vi "create_save_log_file.vi"(0 "Username":string, 1 "Data filepath":path, 2 "Frequency (Hz)":string="280", 3 "Application Directory":string, 5 "Experiment Title":string, 7 "Time constant (ms)":string="100 ms", 9 "Device details":T2={"Device label"="", "Experiment Variable"="", "Variable Value"="", "Pixel"=enum."1"}, 11 "Measurement settings":T1={"Start Wavelength (nm)"=300.0, "End Wavelength (nm)"=900.0, "Increment (nm)"=5.0, "White Bias (No. of Suns)"=1.0, "Averages per wavlength"=1.0, "Time Constant"=8, "Low Pass Filter Slope "=1, "Gain (V/A)"=50.0} {"Gain (V/A)" format="%#.2f"; "Low Pass Filter Slope" items=["6 dB/oct", "12 dB/oct", "18 db/oct", "24 dB/oct"]; "Time Constant" items=["10 us", "30 us", "100 us", "300 us", "1 ms", "3 ms", "10 ms", "30 ms", "100 ms", "300 ms", "1 s", "3 s", "10 s", "30 s", "100 s", "300 s", "1 ks", "3 ks", "10 ks", "30 ks"]; "Averages per wavlength" format="%#.2f"; "White Bias (No. of Suns)" format="%#.2f"; "End Wavelength (nm)" min=350.0 max=1100.0 format="%#.2f"; "Start Wavelength (nm)" min=350.0 max=1100.0 format="%#.2f"}, 12 "Scan number":string, 13 "white bias (# of suns)":dbl, 14 "integrated jsc (mA/cm^2)":dbl) -> (4 "Filepath out":path)   [LabVIEW 2018]
uses:
  typedefs/device_details.ctl
  typedefs/measurement_settings.ctl
  <vilib>/Utility/file.llb/Write Delimited Spreadsheet (string).vi
panel:
  out "file or folder exists?":bool
  in  "headings":string[](array[string])=["timestamp", "device_label", "pixel", "exp_variable", "variable_value", "scan", "start_wl (nm)", "end_wl (nm)", "increment_wl (nm)", "averages_per_wl", "sensitivity", "chopper_freq (Hz)", "time_const", "low-pass_slope (dB)", "white_bias (# suns)", "file_path"]
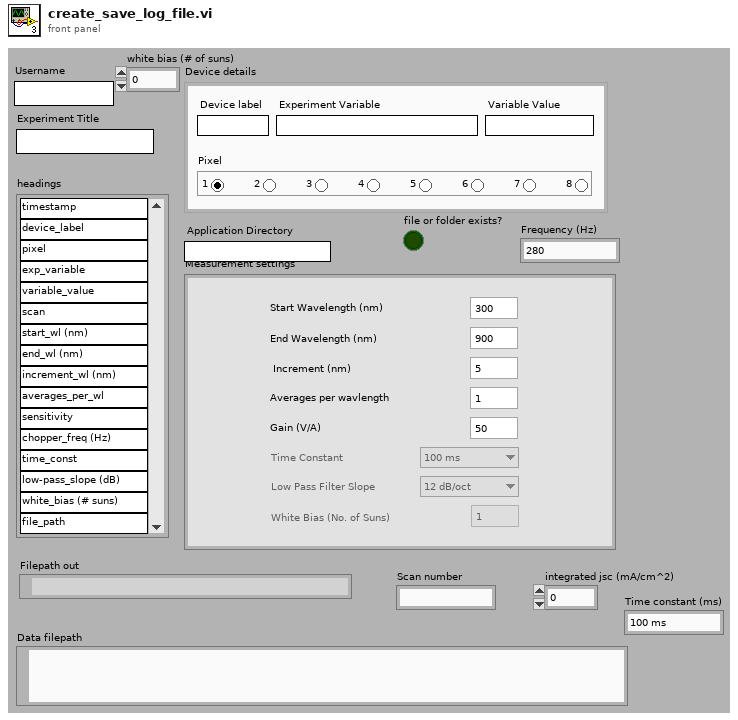
[diagram p1: front panel]
types:
  T1 = typedef "measurement_settings.ctl" = cluster{"Start Wavelength (nm)":dbl, "End Wavelength (nm)":dbl, "Increment (nm)":dbl, "White Bias (No. of Suns)":dbl, "Averages per wavlength":dbl, "Time Constant":u16, "Low Pass Filter Slope ":u16, "Gain (V/A)":dbl}
  T2 = typedef "device_details.ctl" = cluster{"Device label":string, "Experiment Variable":string, "Variable Value":string, "Pixel":enum32{"No Selection", "1", "2", "3", "4", "5", "6", "7", "8"}}
  T3 = enum32{"No Selection", "1", "2", "3", "4", "5", "6", "7", "8"}
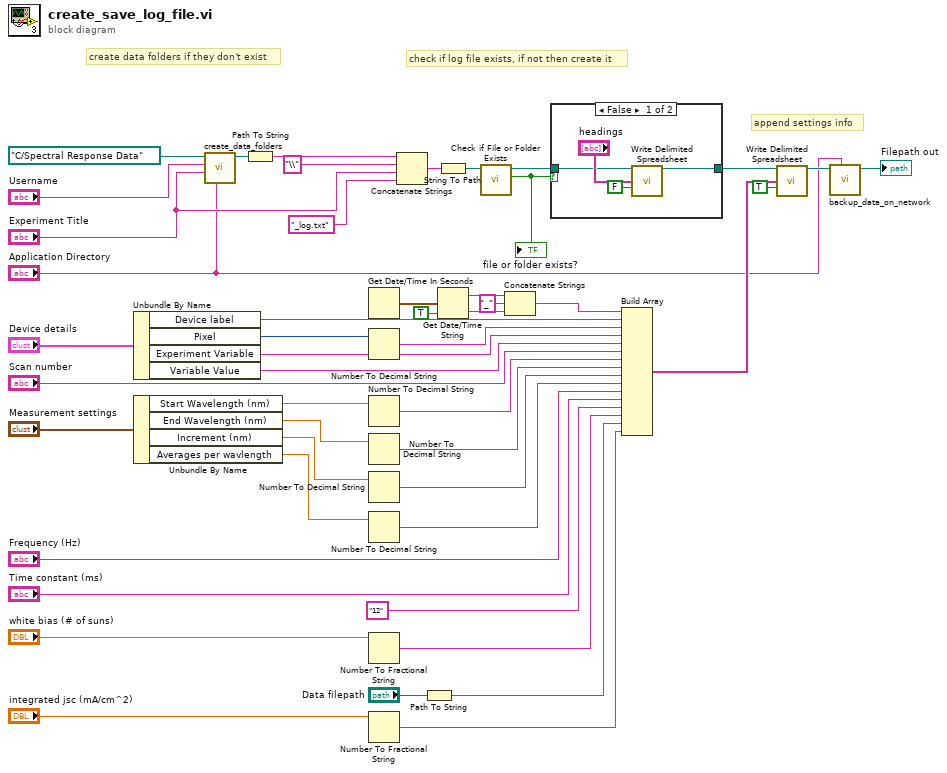
[diagram p0: block diagram]
diagram:
  # "append settings info"
  # "create data folders if they don't exist"
  # "check if log file exists, if not then create it"
  n1 = Unbundle By Name("Device details") -> ("Device label"=w24:string, "Pixel"=w26:T3, "Experiment Variable"=w22:string, "Variable Value"=w21:string)
  n2 = Unbundle By Name("Measurement settings") -> ("Start Wavelength (nm)"=w30:dbl, "End Wavelength (nm)"=w29:dbl, "Increment (nm)"=w28:dbl, "Averages per wavlength"=w27:dbl)
  n3 = call "create_data_folders.vi"("Application Directory"="Application Directory", "Experiment Title"="Experiment Title", "Username"="Username", "Folderpath on C:"=path "C:/Spectral Response Data") -> ("Folderpath on C: out"=w48:path)  [unwired: 7 in]
  n4 = Path To String(path=w48) -> (string=w47:string)
  n5 = Get Date/Time In Seconds() -> (seconds since 1Jan1904=w38:timestamp)
  n6 = Number To Decimal String(number=w26) -> (decimal integer string=w23:string)  [unwired: 1 in]
  n7 = Number To Decimal String(number=w30) -> (decimal integer string=w19:string)  [unwired: 1 in]
  n8 = Number To Decimal String(number=w29) -> (decimal integer string=w18:string)  [unwired: 1 in]
  n9 = Number To Decimal String(number=w28) -> (decimal integer string=w17:string)  [unwired: 1 in]
  n10 = Number To Decimal String(number=w27) -> (decimal integer string=w16:string)  [unwired: 1 in]
  n11 = Number To Fractional String(number="white bias (# of suns)") -> (F-format string=w12:string)  [unwired: 3 in]
  n12 = Number To Fractional String(number="integrated jsc (mA/cm^2)") -> (F-format string=w2:string)  [unwired: 3 in]
  n13 = Concatenate Strings(w47, "\\", "Experiment Title", "_log.txt") -> (w44:string)
  n14 = Path To String(path="Data filepath") -> (string=w10:string)
  n15 = String To Path(string=w44) -> (path=w41:path)
  n16 = Get Date/Time String(seconds (now)=w38, want seconds? (F)=TRUE) -> (date string=w37:string, time string=w35:string)  [unwired: 1 in]
  n17 = call <vilib>:"Check if File or Folder Exists.vi"("path"=w41) -> ("file or folder exists?"=w33:bool, "dup path"=w34:path)  [unwired: 8 in, 1 out]
  "file or folder exists?" <- w33
  n18 = Concatenate Strings(w37, "_" ("string"), w35) -> (w25:string)
  n19 = case shown="False" w33 {
    tunnel: w34 -> [w50 w53]
    tunnel: [w49 w53] -> w9
    frame False {
      n20 = call-poly <vilib>:"Write Delimited Spreadsheet.vi"("file path (dialog if empty)"=w50, "1D data"="headings", "append to file? (new file:F)"=FALSE) -> ("new file path (Not A Path if cancelled)"=w49:path)  [unwired: 11 in, 1 out]
    }
    frame True {
    }
  }
  n21 = Build Array(w25, w24, w23, w22, w21, "Scan number", w19, w18, w17, w16, "Frequency (Hz)", "Time constant (ms)", "12" ("string"), w12, w10, w2) -> (w8:string[])
  n22 = call-poly <vilib>:"Write Delimited Spreadsheet.vi"("file path (dialog if empty)"=w9, "1D data"=w8, "append to file? (new file:F)"=TRUE) -> ("new file path (Not A Path if cancelled)"=w6:path)  [unwired: 11 in, 1 out]
  n23 = call "backup_data_on_network.vi"("Application Directory"="Application Directory", "Filepath in"=w6) -> ("Filepath out"=→"Filepath out":path)  [unwired: 9 in]
